vi "set keypair file.vi"(8 "error in":errorcluster, 9 "key":path, 10 "cert":path, 11 "lvlibretls configurable context in":refnum<class "lvlibretls configurable context.lvclass">) -> (0 "error out":errorcluster, 3 "lvlibretls configurable context out":refnum<class "lvlibretls configurable context.lvclass">)   [LabVIEW 2016, in "lvlibretls configurable context.lvclass"]
uses:
  lvlibretls configurable context.lvclass
  lvlibretls configurable context.lvclass/lvlibretls configurable context.ctl
  lv tls dll.lvlib
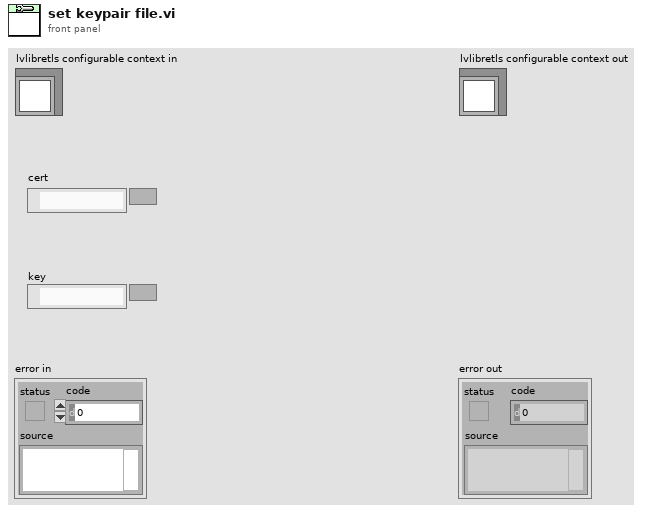
[diagram p1: front panel]
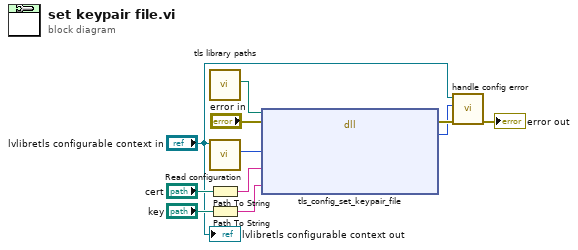
[diagram p0: block diagram]
diagram:
  n1 = call "tls library paths.vi"() -> ("libtls"=w11:path)  [unwired: 8 in, 3 out]
  n2 = call "Read configuration.vi"("lvlibretls configurable context in"="lvlibretls configurable context in") -> ("configuration"=w10:u64)  [unwired: 10 in]
  n3 = Path To String(path="cert") -> (string=w4:string)
  n4 = Path To String(path="key") -> (string=w5:string)
  n5 = dll-call lib="C:/Users/IEUser/Desktop/tlssimple/libtls-15.dll" fn="tls_config_set_keypair_file"(path in=w11, error in="error in", "config"=w10, "certfile"=w4, "keyfile"=w5) -> (error out=w9:errorcluster, "return"=w8:i32)  [unwired: 4 in, 1 out]
  n6 = call "handle config error.vi"("error in"=w9, "return"=w8, "lvlibretls configurable context in"="lvlibretls configurable context in") -> ("error out"=→"error out":errorcluster)  [unwired: 8 in]
  "lvlibretls configurable context out" <- "lvlibretls configurable context in"
